vi "TEST - Wait on VIs Unloaded from Memory.vi"(8 "error in (no error)":errorcluster) -> (0 "error out":errorcluster, 2 "pass":bool)   [LabVIEW 2009]
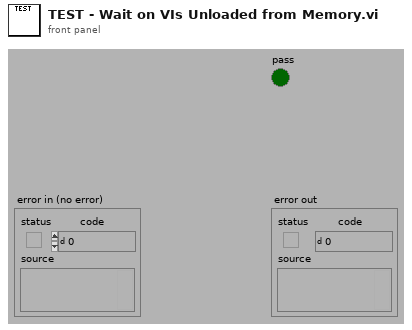
[diagram p1: front panel]
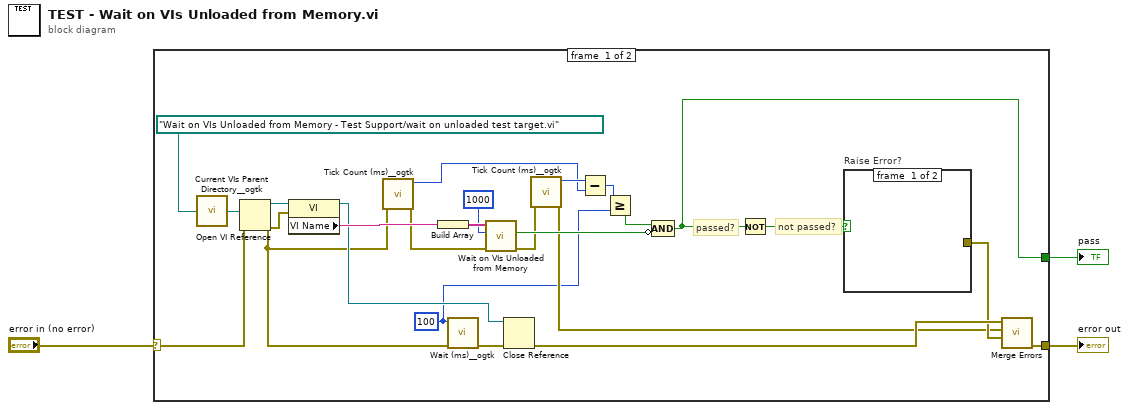
[diagram p0: block diagram]
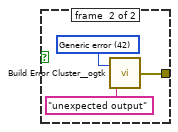
[diagram p2: hidden frame]
diagram:
  n1 = case shown="No Error" "error in (no error)" {
    selector: "error in (no error)" -> [w23 w31]
    tunnel: [w7 _] -> w3
    tunnel: [w27 w31] -> w1
    frame #0 {
      w5 = u32 100 ("milliseconds to wait")
      # "not passed?"
      # "passed?"
      n2 = call <userlib>:"Current VIs Parent Directory__ogtk.vi"("Relative path (.)"=path "Wait on VIs Unloaded from Memory - Test Support/wait on unloaded test target.vi") -> ("Parent Directory (+ Relative)"=w22:path)  [unwired: 4 in]
      n3 = Open VI Reference(vi path=w22, error in (no error)=w23) -> (vi reference=w15:refnum<vi>, error out=w13:errorcluster)  [unwired: 4 in]
      n4 = property class="VI"(reference=w15, error in=w13) -> (reference out=w16:refnum<vi>, "VI Name"=w20:string)  [unwired: 1 out]
      n5 = call <userlib>:"Tick Count (ms)__ogtk.vi"("error in (no error)"=w13) -> ("error out"=w14:errorcluster, "millisecond timer value"=w8:u32)  [unwired: 9 in]
      n6 = Build Array(w20) -> (w19:string[])
      n7 = call <userlib>:"Wait (ms)__ogtk.vi"("error in (no error)"=w13, "milliseconds to wait"=w5) -> ("error out"=w21:errorcluster)  [unwired: 8 in, 1 out]
      n8 = call "Wait on VIs Unloaded from Memory.vi"("error in (no error)"=w14, "ms Timout (100ms)"=u32 1000, "VIs to Wait on"=w19) -> ("error out"=w12:errorcluster, "Timeout?"=w17:bool)  [unwired: 7 in]
      n9 = Close Reference(reference=w16, error in (no error)=w21) -> (error out=w25:errorcluster)
      n10 = call <userlib>:"Tick Count (ms)__ogtk.vi"("error in (no error)"=w12) -> ("error out"=w10:errorcluster, "millisecond timer value"=w9:u32)  [unwired: 9 in]
      n11 = Subtract(x=w9, y=w8) -> (x-y=w6:u32)
      n12 = Greater Or Equal?(x=w6, y=w5) -> (x >= y?=w4:bool)
      n13 = Compound Arithmetic op=AND(w4, invert w17) -> (w7:bool)
      n14 = Not(x=w7) -> (.not. x?=w26:bool)
      n15 = case "Raise Error?" shown="True" w26 {
        tunnel: [_ w28] -> w11
        frame #0 {
        }
        frame #1 {
          w29 = 42 items=["No error", "Argument error", "Memory is full", "Out of zone", "End of file", "File already open", "Generic file I/O error", "File not found", "File permission error", "Disk is full", "Duplicate path", "Too many files open", "System feature not enabled", "Resource file not found", "Cannot add resource", "Resource not found", "Image not found", "Image memory error", "Pen does not exist", "Config type invalid", "Config token not found", "Config parse error", "Config memory error", "Bad external code format", "Bad external code offset", "External code not present", "Null window", "Destroy window error", "Null menu", "Print aborted", "Bad print record", "Print driver error", "Windows error during printing", "Memory error during printing", "Print dialog error", "Generic print error", "Invalid device refnum", "Device not found", "Device parameter error", "Device unit error", "Cannot open device", "Device call aborted", "Generic error", "Cancelled by user", "Object ID too low", "Object ID too high", "Object not in heap", "Unknown heap", "Unknown object (invalid DefProc)", "Unknown object (DefProc not in table)", "Message out of range", "Invalid (null) method", "Unknown message", "Manager call not supported", "Bad address", "Network operation in progress", "Network operation timed out", "Connection is busy", "Network attribute not supported", "Network error", "Address in use", "System out of memory", "Connection aborted", "Connection refused", "Not connected", "Already connected", "Connection closed", "Initialization error (interapplication manager)", "Bad occurrence", "Wait on unbound occurrence handler", "Occurrence queue overflow", "Datalog type conflict", "Unused", "Unrecognized type (interapplication manager)", "Memory corrupt", "Failed to make temporary DLL", "Old CIN version", "Drag socket not found", "Failed to load drop-object", "Failed to register OLE object", "Failed to release OLE object", "Format specifier type mismatch", "Unknown format specifier", "Too few format specifiers", "Too many format specifiers", "Scan failed", "Newer CIN version", "Error converting to variant", "Runtime menu error", "Password tampered", "Variant attribute not found", "Incompatible variant data type", "Event data is not available", "Event Store is not present", "Occurrence is not found", "Event Queue is not created", "Event info is not available", "Refnum passed is NULL", "Error retrieving Class GUID", "Error retrieving CoClass GUID", "Error retrieving TypeLib GUID.", "Bad built application magic bytes.", "Specific driver is different from the specific driver associated with the Logical Name.", "There is no session opened to the class driver.", "Max Error", "MAX - Error with config objects", "MAX - Error loading configuration", "MAX - Group not supported"]
          n16 = call <userlib>:"Build Error Cluster__ogtk.vi"("String to Prepend to source (\"\")"="unexpected output" ("String to Prepend to source (\"\")"), "code"=w29) -> ("error out"=w28:errorcluster)
        }
      }
      n17 = call <vilib>:"Merge Errors.vi"("error in 3 (no error)"=w11, "error in 2 (no error)"=w10, "error in 1 (no error)"=w25) -> ("error out"=w27:errorcluster)  [unwired: 4 in]
    }
    frame #1 {
    }
  }
  "pass" <- w3
  "error out" <- w1
